vi "auto_data.vi"() -> ()   [LabVIEW 2015]
uses:
  vi_execute.ctl
panel:
  in  "hgt_tgt":dbl
  in  "advance":bool
  in  "routine finished":bool
  in  "active step":u8
  in  "auto results":string[](array[string])
  in  "init_done":bool
  in  "auto list":string[](array[string])=["none.bee", "test_1CanAuto.bee", "", "", "", "", "", ""]
  out "command vectors":T1[][](array[typedef])
  in  "auto to run":i8=2
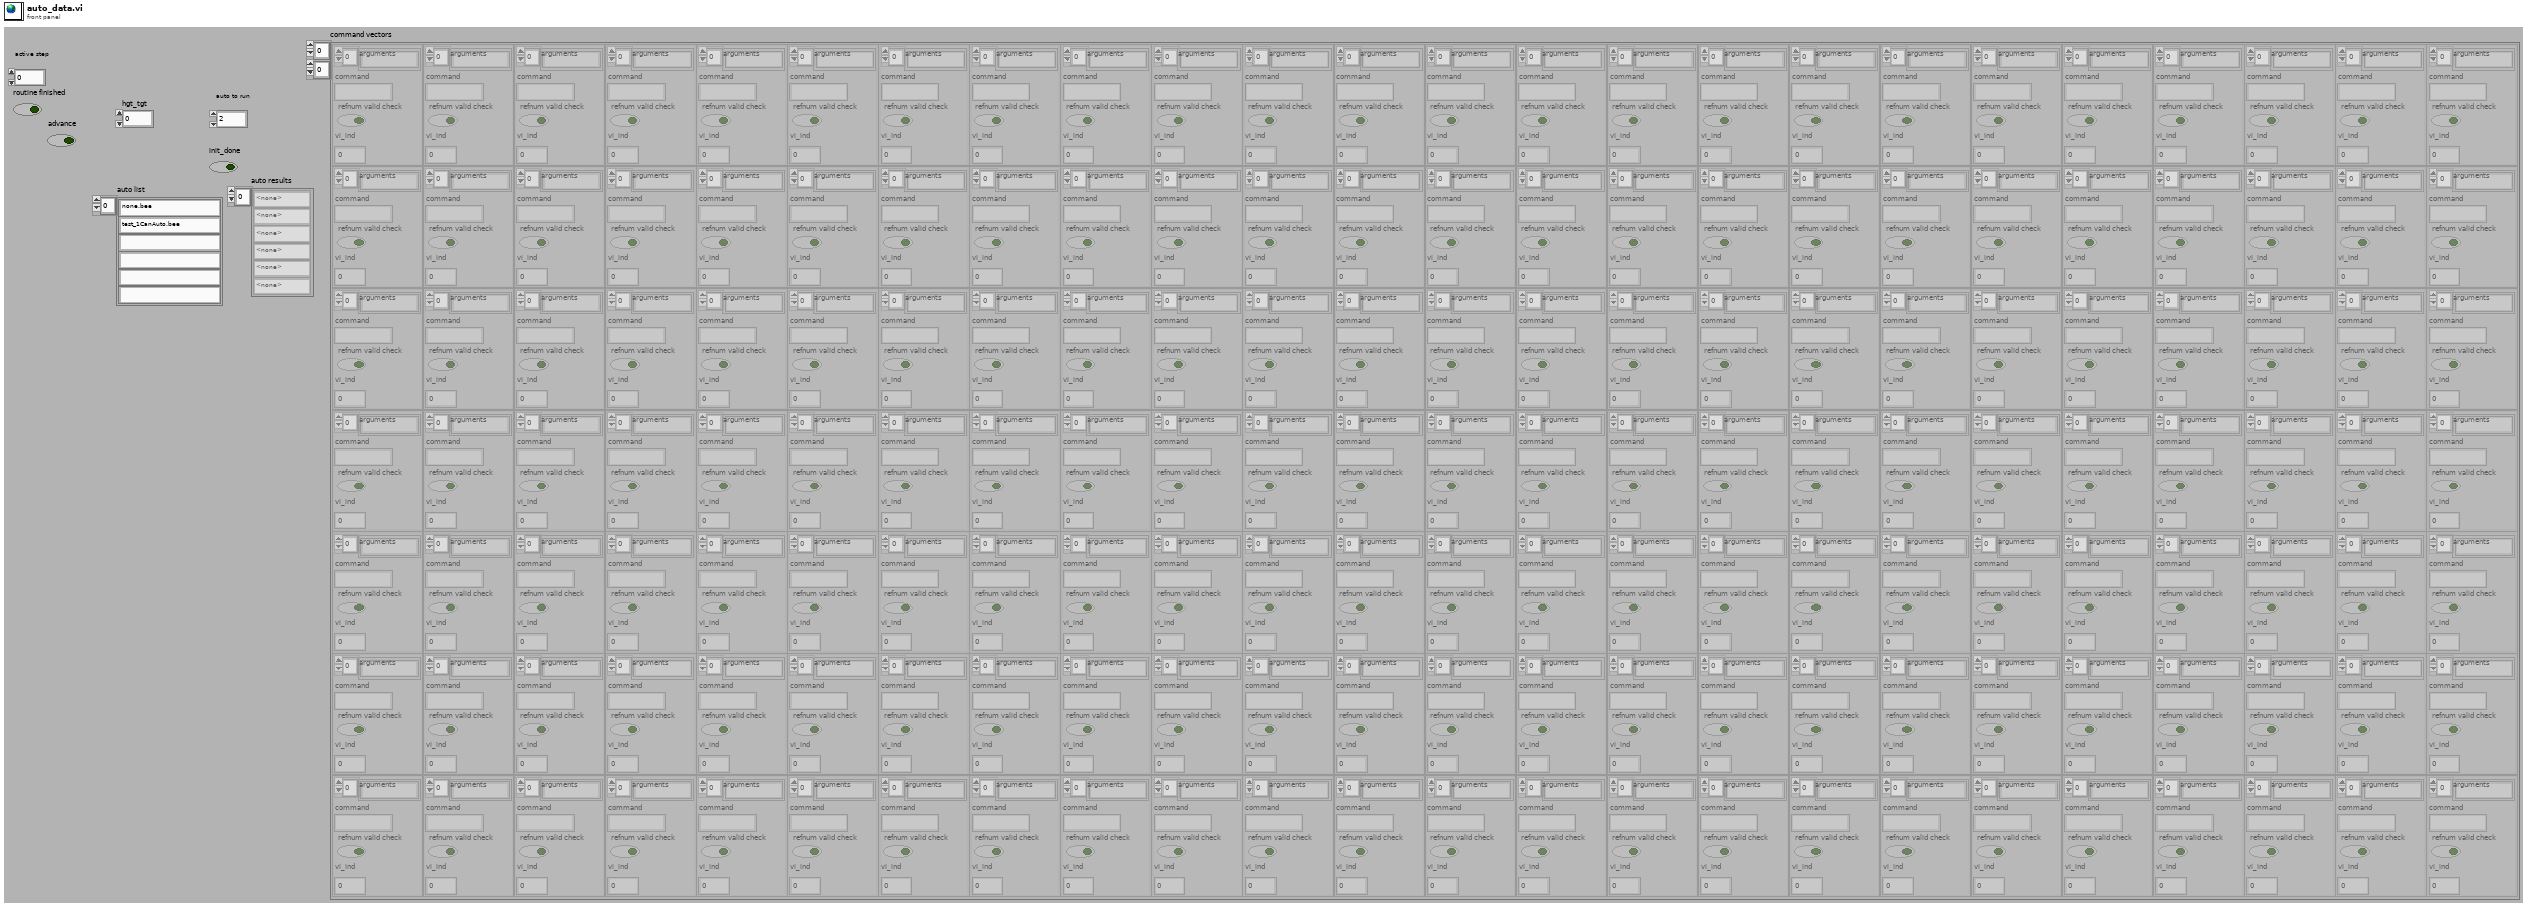
[diagram p1: front panel]
types:
  T1 = typedef "vi_execute.ctl" = cluster{"arguments":string[], "command":string, "refnum valid check":bool, "vi_ind":u8}
diagram:
